vi "FGV - KH Settings.vi"(4 "error in":errorcluster, 6 "Function":enum16{"write", "read"}(ring), 7 "Channel Setting":T1=[{"Channel"=enum."Channel 2", "Gain"=enum."10x", "Shunt Resistor"=enum."50 Ohms", "Input Config"=enum."SE- (+gnd)"}, {"Channel"=enum."Channel 3", "Gain"=enum."1000x", "Shunt Resistor"=enum."50k Ohms", "Input Config"=enum."Differential"}, {"Channel"=enum."Channel 4", "Gain"=enum."1000x", "Shunt Resistor"=enum."50 Ohms", "Input Config"=enum."SE- (+gnd)"}, {"Channel"=enum."Channel 5", "Gain"=enum."1000x", "Shunt Resistor"=enum."50 Ohms", "Input Config"=enum."SE- (+gnd)"}, {"Channel"=enum."Channel 6", "Gain"=enum."1000x", "Shunt Resistor"=enum."50 Ohms", "Input Config"=enum."SE- (+gnd)"}, {"Channel"=enum."Channel 7", "Gain"=enum."1000x", "Shunt Resistor"=enum."50k Ohms", "Input Config"=enum."Differential"}, {"Channel"=enum."Channel 8", "Gain"=enum."1000x", "Shunt Resistor"=enum."50 Ohms", "Input Config"=enum."SE- (+gnd)"}, {"Channel"=enum."Channel 8", "Gain"=enum."1000x", "Shunt Resistor"=enum."50k Ohms", "Input Config"=enum."Differential"}]) -> (0 "error out":errorcluster, 3 "Channel Setting 2":T1)   [LabVIEW 2016, in "Instrument.KH7008.lvclass"]
uses:
  Instrument.KH7008.lvclass
  typedefs/KH_control_array.ctl
  typedefs/KH_control.ctl
  typedefs/Channel-Enum.ctl
  typedefs/Gain-Enum.ctl
  typedefs/Shunt-Enum.ctl
  typedefs/Input Configuration-Enum.ctl
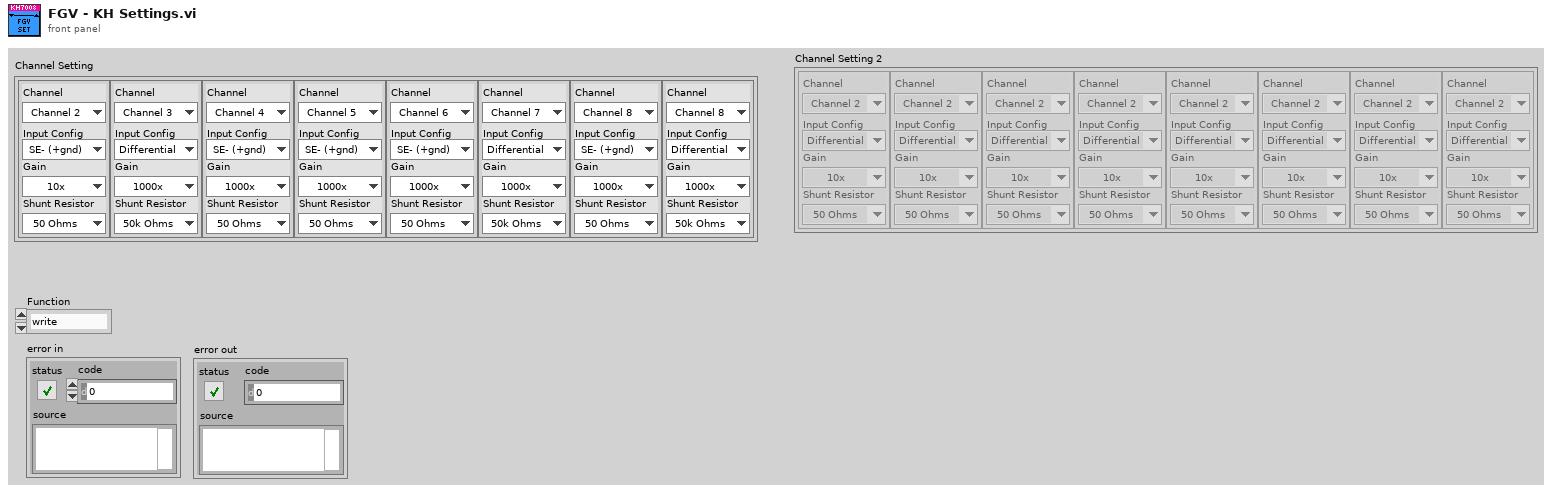
[diagram p1: front panel]
types:
  T1 = typedef "Instrument.KH7008.lvclass/KH_control_array.ctl" = T2[]
  T2 = typedef "Instrument.KH7008.lvclass/KH_control.ctl" = cluster{"Channel":T3, "Gain":T4, "Shunt Resistor":T5, "Input Config":T6}
  T3 = typedef "Instrument.KH7008.lvclass/Channel-Enum.ctl" = enum16{"Channel 1", "Channel 2", "Channel 3", "Channel 4", "Channel 5", "Channel 6", "Channel 7", "Channel 8"}
  T4 = typedef "Instrument.KH7008.lvclass/Gain-Enum.ctl" = enum16{"1x", "10x", "100x", "1000x"}
  T5 = typedef "Instrument.KH7008.lvclass/Shunt-Enum.ctl" = enum16{"Open", "50 Ohms", "500 Ohms", "5k Ohms", "50k Ohms"}
  T6 = typedef "Instrument.KH7008.lvclass/Input Configuration-Enum.ctl" = enum16{"Ground", "SE+ (-gnd)", "SE- (+gnd)", "Differential"}
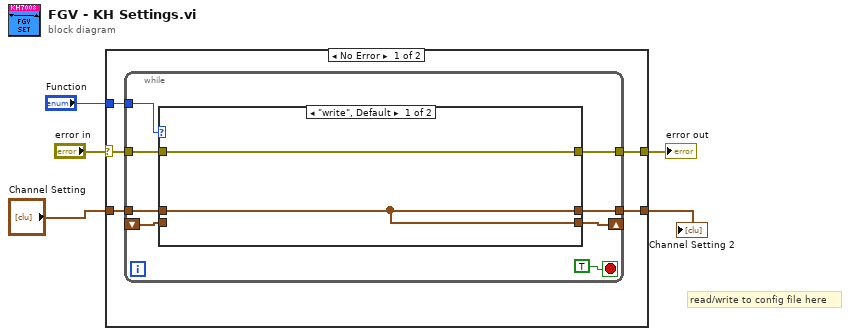
[diagram p0: block diagram]
diagram:
  # "read/write to config file here"
  n1 = case shown="No Error" "error in" {
    selector: "error in" -> [w10 w24]
    tunnel: [w9 w24] -> w4
    tunnel: "Channel Setting" -> [w8 w23]
    tunnel: [w7 w23] -> w2
    tunnel: "Function" -> [w6 _]
    frame No Error {
      n2 = while {
        shift-right: [w12] -> _
        shift-left: _ -> [w11]
        tunnel: w10 -> [w17]
        tunnel: [w16] -> w9
        tunnel: w8 -> [w15]
        tunnel: [w14] -> w7
        tunnel: w6 -> [w13]
        stop <- TRUE stop-if-true
        n3 = case shown="\"write\", Default" w13 {
          tunnel: w17 -> [w20 w22]
          tunnel: [w20 w22] -> w16
          tunnel: w15 -> [w19 _]
          tunnel: [w19 w21] -> w14
          tunnel: [w19 w21] -> w12
          tunnel: w11 -> [_ w21]
          frame "write", Default {
          }
          frame "read" {
          }
        }
      }
    }
    frame Error {
    }
  }
  "error out" <- w4
  "Channel Setting 2" <- w2
